vi "Enque Epics Message Int.vi"(0 "Queue in":refnum<queue>, 1 "Message":string, 2 "UInt32":u32, 3 "error in (no error)":errorcluster, 4 "Boolean":bool) -> (9 "error out":errorcluster)   [LabVIEW 2014]
uses:
  Message Queue/Message Cluster.ctl
  Message Queue/Message Queue.lvlib
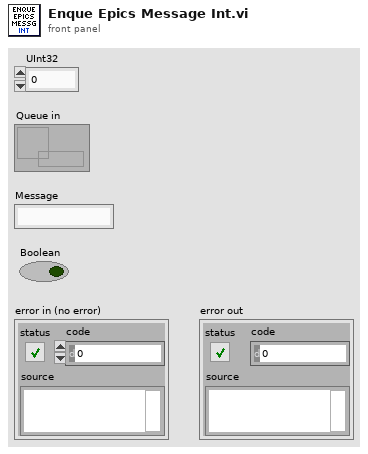
[diagram p1: front panel]
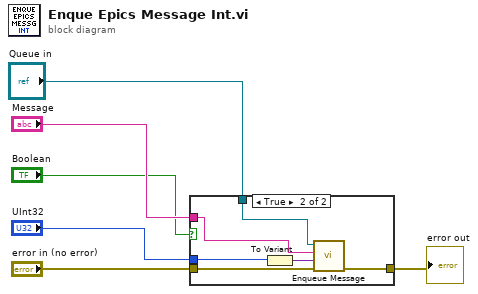
[diagram p0: block diagram]
diagram:
  n1 = case shown="True" "Boolean" {
    tunnel: "error in (no error)" -> [w7 w13]
    tunnel: [w7 w12] -> w3
    tunnel: "Queue in" -> [_ w11]
    tunnel: "UInt32" -> [_ w9]
    tunnel: "Message" -> [_ w8]
    frame False {
    }
    frame True {
      n2 = To Variant(anything=w9) -> (Variant=w10:variant)
      n3 = call "Enqueue Message.vi"("error in (no error)"=w13, "Message Data"=w10, "Message"=w8, "Message Queue"=w11) -> ("error out"=w12:errorcluster)  [unwired: 6 in, 1 out]
    }
  }
  "error out" <- w3
